vi "Load .net control.vi"() -> (0 "GetHashCode":i32, 1 "source":string, 2 "Enabled":bool)   [LabVIEW 2013]
uses:
  C:/builds/Untitled Project 1/My Source Distribution/Thorlabs.MotionControl.Tools.WPF.UI.dll
  Thorlabs.MotionControl.Tools.WPF.UI.dll
  C:/builds/Untitled Project 1/My Source Distribution/Thorlabs.MotionControl.Controls.dll
  Thorlabs.MotionControl.Controls.dll
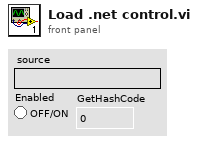
[diagram p1: front panel]
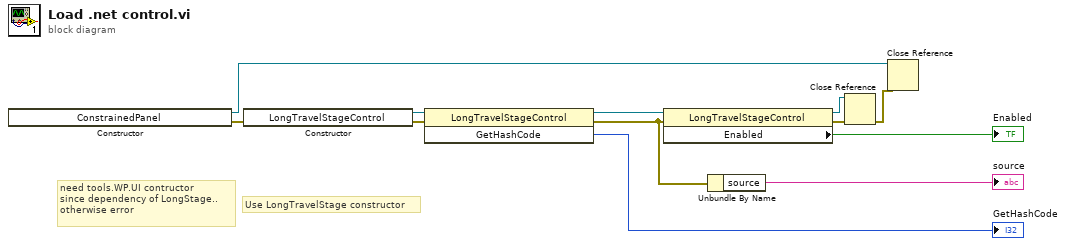
[diagram p0: block diagram]
diagram:
  # "need tools.WP.UI contructor \nsince dependency of LongStage..\notherwise error"
  # "Use LongTravelStage constructor"
  n1 = constructor class="Thorlabs.MotionControl.Tools.WP"() -> (reference out=w5:refnum<k24>, error out=w4:errorcluster)  [unwired: 3 in, 1 out]
  n2 = constructor class="LongTravelStageControl"(error in=w4) -> (reference out=w12:refnum<k24>, error out=w10:errorcluster)  [unwired: 2 in, 1 out]
  n3 = invoke class="LongTravelStageControl" method="GetHashCode"(reference=w12, error in=w10) -> (reference out=w9:refnum<k24>, error out=w3:errorcluster, "GetHashCode"=→"GetHashCode":i32)  [unwired: 1 in]
  n4 = property class="LongTravelStageControl"(reference=w9, error in=w3) -> (reference out=w8:refnum<k24>, error out=w2:errorcluster, "Enabled"=→"Enabled":bool)
  n5 = Unbundle By Name(w3) -> ("source"=→"source":string)
  n6 = Close Reference(reference=w8, error in (no error)=w2) -> (error out=w1:errorcluster)
  n7 = Close Reference(reference=w5, error in (no error)=w1) -> ()  [unwired: 1 out]
